vi "test.ingest_csv.vi"   [LabVIEW 2020]
uses:
  datasources/dataset/dataset.lvclass
  datasources/dataset/dataset.lvclass/dataset.ctl
  Nominal Client/Nominal Client.lvclass/Nominal Client.ctl
  nominal types/workspace/workspace.lvclass/workspace.ctl
  81c5314d-0c17-4e40-9591-806fc92e59be.vi
  40e2c779-94f0-4ff6-913c-6196809b7e71.vi
  datasources/dataset/datasetName.set.vi
  Nominal Client/private_data.set.vi
  nominal types/workspace/id.get.vi
  nominal types/workspace/rid.get.vi
  <vilib>/AdvancedString/1D String Array to Delimited String.vi
  Nominal Client/workspace.set.vi
  datasources/gcs/gcs.lvclass
  C:/code/labview-client/lv_src/datasources/source/source.lvclass
  datasources/s3/s3.lvclass
  datasources/source/create_s3.vi
  datasources/target/create_from_existing.vi
  datasources/source/create_gcs.vi
  <vilib>/Utility/file.llb/Application Directory.vi
  <vilib>/Utility/error.llb/Error Cluster From Error Code.vi
  Nominal Client/Palette Items/who_am_i.vi
  datasources/target/create_new.vi
  ts.iso8601/build.iso8601.vi
  ts.relative/build.relative.vi
  Nominal Client/ingest_csv.vi
  Nominal Client/workspace_cache.get_from_rid.vi
  Nominal Client/workspace_cache.get.vi
  User/User.lvclass
  Nominal Client/Nominal Client.lvclass
  nominal types/workspace/workspace.lvclass
  submodules/reqwest-labview/lv-src/reqwest/reqwest.lvclass
  datasources/source/source.lvclass
  timestampMetadata/timestampMetadata.lvclass
  datasources/target/target.lvclass
  nominal types/channelConfig/channelConfig.lvclass
  ts.iso8601/ts.iso8601.lvclass
  ts.relative/ts.relative.lvclass
  nominal types/properties/properties.lvclass
  C:/code/labview-client/lv_src/datasources/payload/payload.lvclass
  C:/code/labview-client/lv_src/datasources/s3/s3.lvclass
  C:/code/labview-client/lv_src/datasources/gcs/gcs.lvclass
types:
  T1 = cluster{"channelPrefix":string, "tagKeysFromColumns":string[], "tagColums":map{string, string}, "additionalFileTags":map{string, string}}
  T2 = enum16{"DAYS", "HOURS", "MINUTES", "SECONDS", "MILLISECONDS", "MICROSECONDS", "NANOSECONDS", "PICOSECONDS"}
  T3 = cluster{"dataset":refnum<class "dataset.lvclass">, "channelConfig":refnum<class "channelConfig.lvclass">}
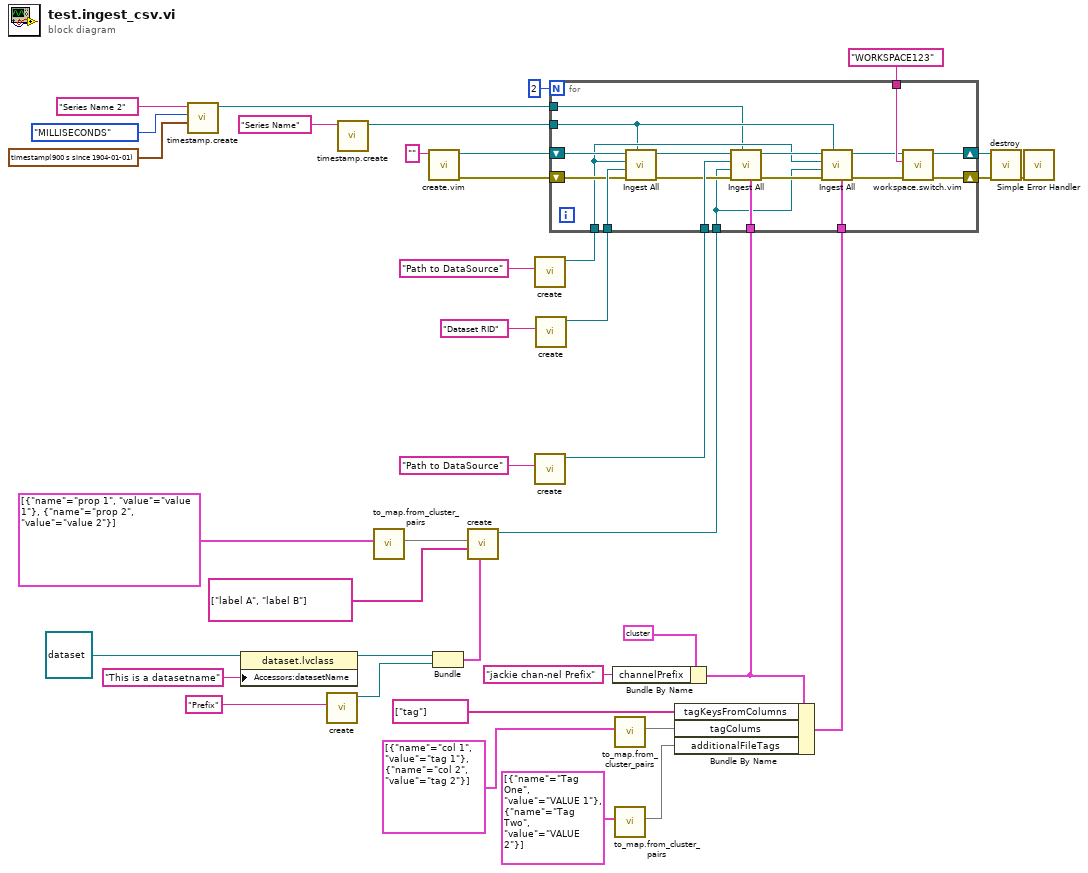
[diagram p0: block diagram]
diagram:
  n1 = call-poly "timestamp.create.vi"("Offset"=timestamp(900 s since 1904-01-01), "Time Unit"=T2."MILLISECONDS", "Time Series Name"="Series Name 2" ("seriesName")) -> ("Timestamp Metadata"=w26:refnum<class "timestampMetadata.lvclass">)  [unwired: 8 in]
  n2 = property class="dataset.lvclass"(reference=refnum<class "dataset.lvclass"> refnum ("dataset"), "Accessors:datasetName"="This is a datasetname" ("datasetName")) -> (reference out=w31:refnum<class "dataset.lvclass">)  [unwired: 1 in, 1 out]
  n3 = call "create.vi"("prefixTreeDelimiter"="Prefix") -> ("channelConfig"=w10:refnum<class "channelConfig.lvclass">)  [unwired: 10 in]
  n4 = call-poly "timestamp.create.vi"("seriesName"="Series Name") -> ("Timestamp Metadata"=w29:refnum<class "timestampMetadata.lvclass">)  [unwired: 10 in]
  n5 = call "to_map.from_cluster_pairs.vi"("properties (cluster pairs)"=cluster{"name":string, "value":string}[] [{"name"="prop 1", "value"="value 1"}, {"name"="prop 2", "value"="value 2"}] ("properties")) -> ("properties (map)"=w5:map{string, string})  [unwired: 10 in]
  n6 = call "create.vim"("API Token (string or path)"="") -> ("error out"=w35:errorcluster, "Nominal Client"=w36:refnum<class "Nominal Client.lvclass">)  [unwired: 8 in, 1 out]
  n7 = Bundle("dataset"=w31, "channelConfig"=w10) -> (w12:T3)  [unwired: 1 in]
  n8 = call-poly "create.vi"("Optional"=w12, "Labels"=string[] ["label A", "label B"] ("labels"), "Properties"=w5) -> ("New Target"=w13:refnum<class "target.lvclass">)  [unwired: 8 in]
  n9 = call-poly "create.vi"("Path"="Path to DataSource") -> ("source"=w18:refnum<class "s3.lvclass">)  [unwired: 10 in]
  n10 = call-poly "create.vi"("Path"="Path to DataSource") -> ("source"=w14:refnum<class "gcs.lvclass">)  [unwired: 10 in]
  n11 = call-poly "create.vi"("dataset RID"="Dataset RID" ("RID")) -> ("Existing Target"=w16:refnum<class "target.lvclass">)  [unwired: 10 in]
  n12 = Bundle By Name(cluster=T1 {"channelPrefix"="", "tagKeysFromColumns"=[], "tagColums"={}, "additionalFileTags"={}} ("optional"), "channelPrefix"="jackie chan-nel Prefix") -> (w21:T1)
  n13 = call "to_map.from_cluster_pairs.vi"("properties (cluster pairs)"=cluster{"name":string, "value":string}[] [{"name"="col 1", "value"="tag 1"}, {"name"="col 2", "value"="tag 2"}] ("properties")) -> ("properties (map)"=w2:map{string, string})  [unwired: 10 in]
  n14 = call "to_map.from_cluster_pairs.vi"("properties (cluster pairs)"=cluster{"name":string, "value":string}[] [{"name"="Tag One", "value"="VALUE 1"}, {"name"="Tag Two", "value"="VALUE 2"}] ("properties")) -> ("properties (map)"=w3:map{string, string})  [unwired: 10 in]
  n15 = Bundle By Name(cluster=w21, "tagKeysFromColumns"=string[] ["tag"] ("labels"), "tagColums"=w2, "additionalFileTags"=w3) -> (w20:T1)
  n16 = for {
    N: 2 -> [_]
    tunnel: w16 -> [w58]
    tunnel: w18 -> [w44]
    tunnel: w14 -> [w57]
    tunnel: w13 -> [w43]
    shift-right: [w52] -> w37
    shift-left: w35 -> [w54]
    shift-right: [w51] -> w39
    shift-left: w36 -> [w53]
    tunnel: "WORKSPACE123" ("RID") -> [w50]
    tunnel: w29 -> [w41]
    tunnel: w26 -> [w40]
    tunnel: w21 -> [w49]
    tunnel: w20 -> [w42]
    n17 = call-poly "Ingest All.vi"("timestampMetadata"=w41, "error in"=w54, "Target"=w58, "Source"=w44, "Nominal Client in"=w53) -> ("error out"=w55:errorcluster, "Nominal Client out"=w56:refnum<class "Nominal Client.lvclass">)  [unwired: 3 in, 2 out]
    n18 = call-poly "Ingest All.vi"("optional"=w49, "timestampMetadata"=w40, "error in"=w55, "Target"=w43, "Source"=w57, "Nominal Client in"=w56) -> ("error out"=w48:errorcluster, "Nominal Client out"=w47:refnum<class "Nominal Client.lvclass">)  [unwired: 2 in, 2 out]
    n19 = call-poly "Ingest All.vi"("optional"=w42, "timestampMetadata"=w41, "error in"=w48, "Target"=w43, "Source"=w44, "Nominal Client in"=w47) -> ("error out"=w46:errorcluster, "Nominal Client out"=w45:refnum<class "Nominal Client.lvclass">)  [unwired: 2 in, 2 out]
    n20 = call "workspace.switch.vim"("error in"=w46, "Workspace (Object, RID, Path)"=w50, "Nominal Client in"=w45) -> ("error out"=w52:errorcluster, "Nominal Client out"=w51:refnum<class "Nominal Client.lvclass">)  [unwired: 7 in]
  }
  n21 = call "destroy.vi"("error in"=w37, "Nominal Client"=w39) -> ("error out"=w23:errorcluster)  [unwired: 9 in]
  n22 = call <vilib>:"Simple Error Handler.vi"("error in (no error)"=w23) -> ()  [unwired: 4 in, 5 out]
